vi "Argument check.vi"(8 "error in":errorcluster, 10 "Arg":string="supint->out2,12", 11 "par":string="export void vtSysPwrSupVoltSet (char vt7001CfgEntry[], float volt)") -> (0 "error out":errorcluster, 3 "Check result":string="√")   [LabVIEW 2010]
panel:
  out "Enum":T1(ring)=enum."float"
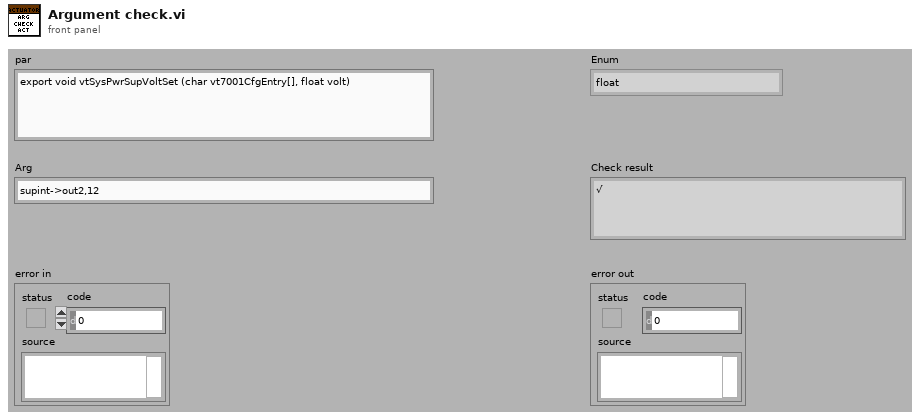
[diagram p1: front panel]
types:
  T1 = enum16{"char", "float", "double", "int", "long", "enum"}
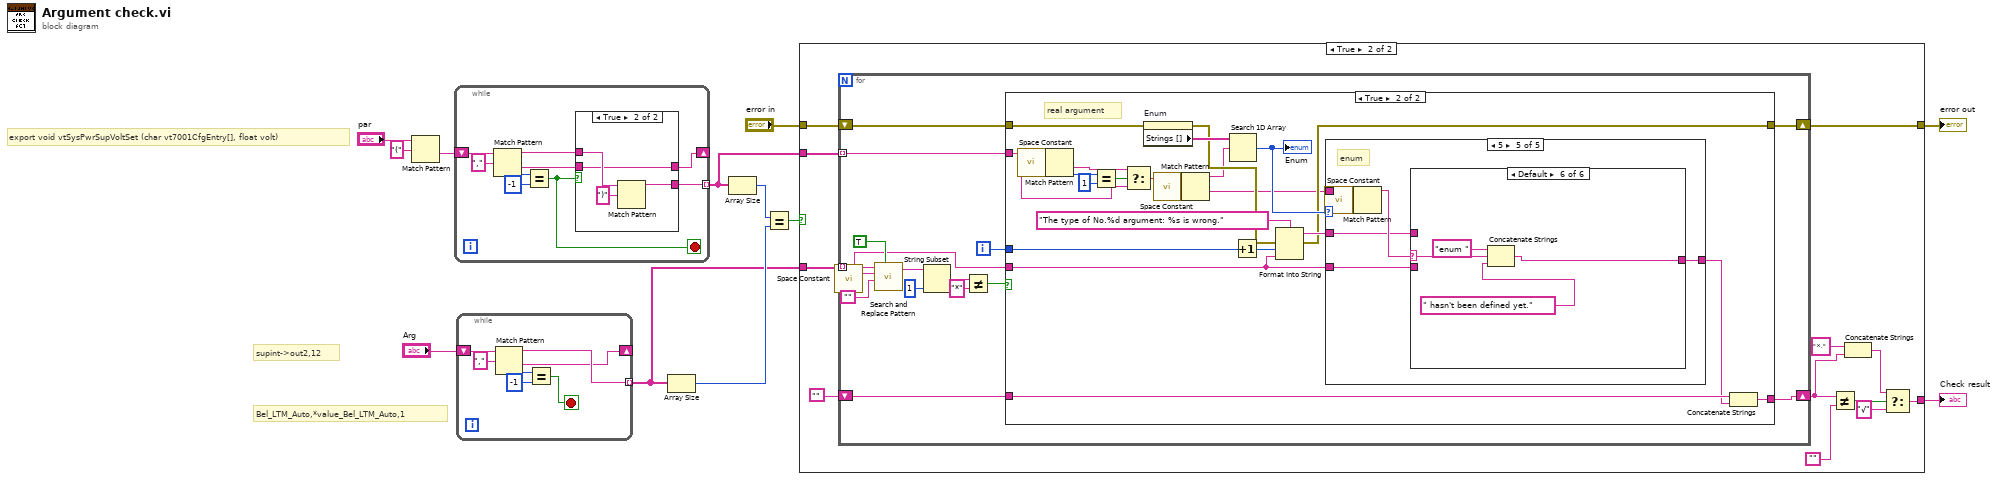
[diagram p0: block diagram]
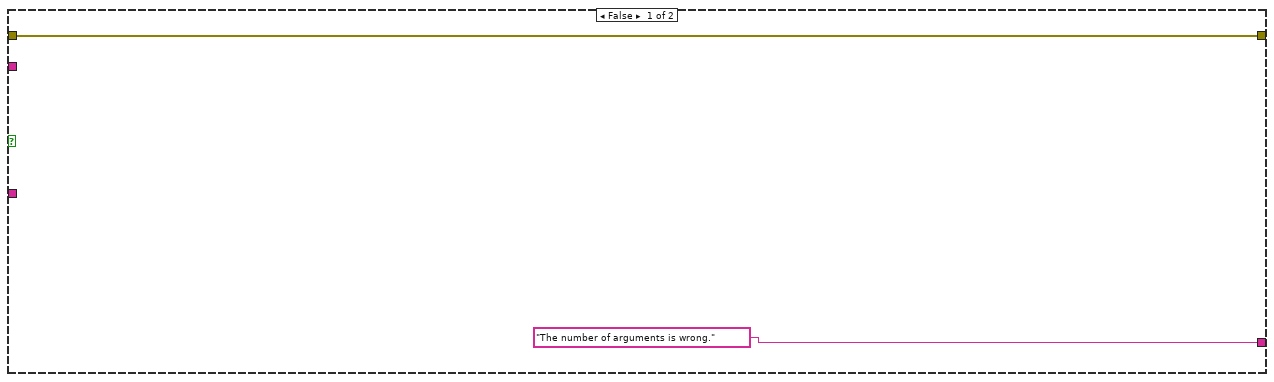
[diagram p2: hidden frame]
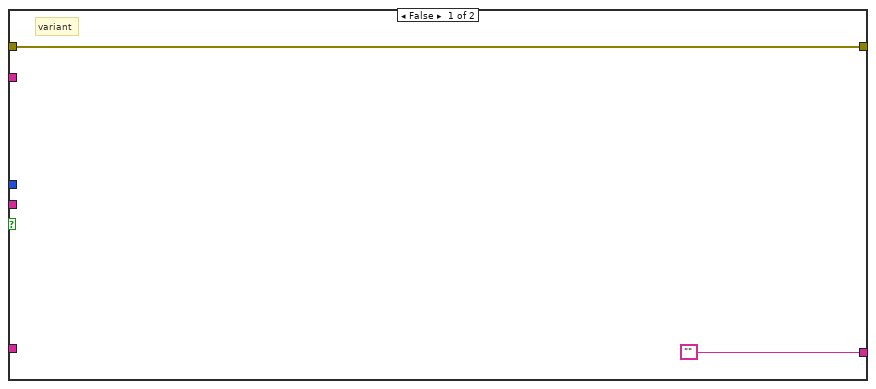
[diagram p3: hidden frame]
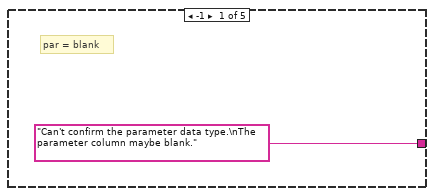
[diagram p4: hidden frame]
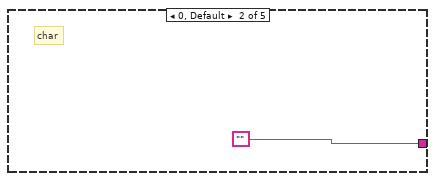
[diagram p5: hidden frame]
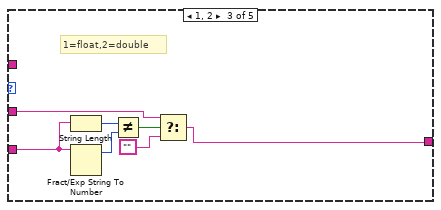
[diagram p6: hidden frame]
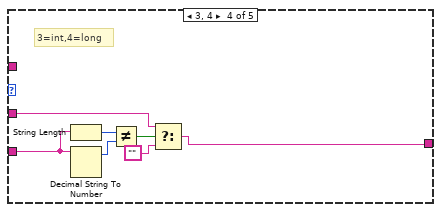
[diagram p7: hidden frame]
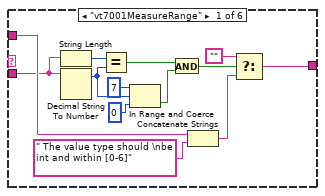
[diagram p8: hidden frame]
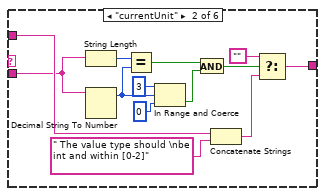
[diagram p9: hidden frame]
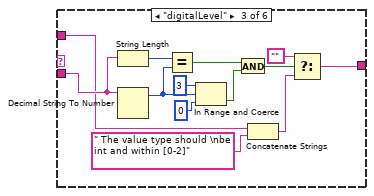
[diagram p10: hidden frame]
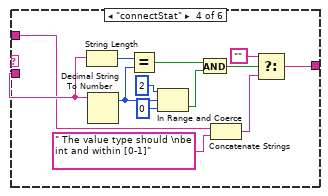
[diagram p11: hidden frame]
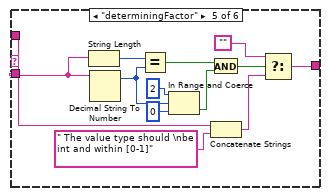
[diagram p12: hidden frame]
diagram:
  # "Bel_LTM_Auto,*value_Bel_LTM_Auto,1"
  # "supint->out2,12"
  # "export void vtSysPwrSupVoltSet (char vt7001CfgEntry[], float volt)"
  n1 = Match Pattern(string="par", regular expression="(") -> (after substring=w11:string)  [unwired: 1 in, 3 out]
  n2 = while {
    shift-right: [w14] -> _
    shift-left: w11 -> [w21]
    tunnel: [w16] -> w7 mode=indexing
    stop <- w13 stop-if-true
    n3 = Match Pattern(string=w21, regular expression=",") -> (before substring=w17:string, after substring=w15:string, offset past match=w19:i32)  [unwired: 1 in, 1 out]
    n4 = Equal?(x=w19, y=-1) -> (x = y?=w13:bool)
    n5 = case shown="True" w13 {
      tunnel: w17 -> [w23 w27]
      tunnel: [w23 w25] -> w16
      tunnel: w15 -> [w22 w24]
      tunnel: [w22 w24] -> w14
      frame False {
      }
      frame True {
        n6 = Match Pattern(string=w27, regular expression=")") -> (before substring=w25:string)  [unwired: 1 in, 3 out]
      }
    }
  }
  n7 = while {
    shift-right: [w29] -> _
    shift-left: "Arg" -> [w34]
    tunnel: [w30] -> w6 mode=indexing
    stop <- w28 stop-if-true
    n8 = Match Pattern(string=w34, regular expression=",") -> (before substring=w30:string, after substring=w29:string, offset past match=w32:i32)  [unwired: 1 in, 1 out]
    n9 = Equal?(x=w32, y=-1) -> (x = y?=w28:bool)
  }
  n10 = Array Size(array=w6) -> (size(s)=w9:i32)
  n11 = Array Size(array=w7) -> (size(s)=w10:i32)
  n12 = Equal?(x=w10, y=w9) -> (x = y?=w8:bool)
  n13 = case shown="True" w8 {
    tunnel: w7 -> [_ w48]
    tunnel: w6 -> [_ w47]
    tunnel: ["The number of arguments is wrong." w42] -> w5
    tunnel: "error in" -> [w35 w41]
    tunnel: [w35 w40] -> w2
    frame False {
    }
    frame True {
      n14 = for {
        tunnel: w48 -> [w63] mode=indexing
        tunnel: w47 -> [w49] mode=indexing
        shift-right: [w61] -> w38
        shift-left: "" -> [w62]
        shift-right: [w59] -> w40
        shift-left: w41 -> [w60]
        i -> [w50]
        n15 = call <vilib>:"Space Constant.vi"() -> ("String"=w58:string)
        n16 = call <vilib>:"Search and Replace Pattern.vi"("string"=w49, "regular expression (\"\")"=w58, "replace string (\"\")"="", "replace all? (F)"=TRUE) -> ("result string"=w55:string)  [unwired: 1 in, 1 out]
        n17 = String Subset(string=w55, length (rest)=1 ("length (rest)")) -> (substring=w53:string)  [unwired: 1 in]
        n18 = Not Equal?(x=w53, y="*") -> (x != y?=w51:bool)
        n19 = case shown="True" w51 {
          tunnel: w63 -> [_ w82]
          tunnel: w62 -> [_ w74]
          tunnel: ["" w72] -> w61
          tunnel: w60 -> [w64 w71]
          tunnel: [w64 w70] -> w59
          tunnel: w50 -> [_ w69]
          tunnel: w49 -> [_ w68]
          frame False {
            # "variant"
          }
          frame True {
            # "real argument"
            n20 = call <vilib>:"Space Constant.vi"() -> ("String"=w88:string)
            n21 = Match Pattern(string=w82, regular expression=w88) -> (after substring=w86:string, offset past match=w81:i32)  [unwired: 1 in, 2 out]
            n22 = Equal?(x=w81, y=1) -> (x = y?=w87:bool)
            n23 = Select(t=w86, s=w87, f=w82) -> (s? t:f=w83:string)
            n24 = property on="Enum" class="Enum (strict)"(error in=w71) -> (error out=w76:errorcluster, "Strings []"=w84:string[])  [unwired: 1 in, 1 out]
            n25 = call <vilib>:"Space Constant.vi"() -> ("String"=w85:string)
            n26 = Match Pattern(string=w83, regular expression=w85) -> (before substring=w67:string, after substring=w66:string)  [unwired: 1 in, 2 out]
            n27 = Search 1D Array(1D array=w84, element=w67) -> (index of element=w79:i32)  [unwired: 1 in]
            "Enum" <- w79
            n28 = Increment(x=w69) -> (x+1=w77:i32)
            n29 = Format Into String(format string="The type of No.%d argument: %s is wrong.", error in=w76, w77, w68) -> (resulting string=w75:string, error out=w70:errorcluster)  [unwired: 1 in]
            n30 = case shown="5" w79 {
              tunnel: w68 -> [_ _ w95 w104 w106]
              tunnel: w75 -> [_ _ w92 w100 w107]
              tunnel: ["Can't confirm the parameter data type.\nThe parameter column maybe blank." "" w91 w98 w105] -> w73
              tunnel: w66 -> [_ _ _ _ w110]
              frame -1 {
                # "par = blank"
              }
              frame 0, Default {
                # "char"
              }
              frame 1, 2 {
                # "1=float,2=double"
                n31 = String Length(string=w95) -> (length=w97:i32)
                n32 = Fract/Exp String To Number(string=w95) -> (offset past number=w96:i32)  [unwired: 3 in, 1 out]
                n33 = Not Equal?(x=w97, y=w96) -> (x != y?=w94:bool)
                n34 = Select(t=w92, s=w94, f="") -> (s? t:f=w91:string)
              }
              frame 3, 4 {
                # "3=int,4=long"
                n35 = String Length(string=w104) -> (length=w103:i32)
                n36 = Decimal String To Number(string=w104) -> (offset past number=w102:i32)  [unwired: 2 in, 1 out]
                n37 = Not Equal?(x=w103, y=w102) -> (x != y?=w101:bool)
                n38 = Select(t=w100, s=w101, f="") -> (s? t:f=w98:string)
              }
              frame 5 {
                # "enum"
                n39 = call <vilib>:"Space Constant.vi"() -> ("String"=w109:string)
                n40 = Match Pattern(string=w110, regular expression=w109) -> (before substring=w108:string)  [unwired: 1 in, 3 out]
                n41 = case shown="Default" w108 {
                  selector: w108 -> [_ _ _ _ _ w179]
                  tunnel: w107 -> [w113 w126 w138 w151 w164 _]
                  tunnel: w106 -> [w112 w125 w139 w152 w166 _]
                  tunnel: [w111 w124 w137 w150 w165 w177] -> w105
                  frame "vt7001MeasureRange" {
                    n42 = String Length(string=w112) -> (length=w123:i32)
                    n43 = Decimal String To Number(string=w112) -> (offset past number=w121:i32)  [unwired: 2 in, 1 out]
                    n44 = Equal?(x=w123, y=w121) -> (x = y?=w122:bool)
                    n45 = In Range and Coerce(upper limit=7, x=w121, lower limit=0) -> (In Range?=w118:bool)  [unwired: 1 out]
                    n46 = And(x=w122, y=w118) -> (x .and. y?=w117:bool)
                    n47 = Concatenate Strings(w113, " The value type should \nbe int and within [0-6]" ("string")) -> (w115:string)
                    n48 = Select(t="", s=w117, f=w115) -> (s? t:f=w111:string)
                  }
                  frame "currentUnit" {
                    n49 = String Length(string=w125) -> (length=w136:i32)
                    n50 = Decimal String To Number(string=w125) -> (offset past number=w134:i32)  [unwired: 2 in, 1 out]
                    n51 = Equal?(x=w136, y=w134) -> (x = y?=w135:bool)
                    n52 = In Range and Coerce(upper limit=3, x=w134, lower limit=0) -> (In Range?=w131:bool)  [unwired: 1 out]
                    n53 = And(x=w135, y=w131) -> (x .and. y?=w130:bool)
                    n54 = Concatenate Strings(w126, " The value type should \nbe int and within [0-2]" ("string")) -> (w128:string)
                    n55 = Select(t="", s=w130, f=w128) -> (s? t:f=w124:string)
                  }
                  frame "digitalLevel" {
                    n56 = String Length(string=w139) -> (length=w149:i32)
                    n57 = Decimal String To Number(string=w139) -> (offset past number=w147:i32)  [unwired: 2 in, 1 out]
                    n58 = Equal?(x=w149, y=w147) -> (x = y?=w148:bool)
                    n59 = In Range and Coerce(upper limit=3, x=w147, lower limit=0) -> (In Range?=w144:bool)  [unwired: 1 out]
                    n60 = And(x=w148, y=w144) -> (x .and. y?=w143:bool)
                    n61 = Concatenate Strings(w138, " The value type should \nbe int and within [0-2]" ("string")) -> (w141:string)
                    n62 = Select(t="", s=w143, f=w141) -> (s? t:f=w137:string)
                  }
                  frame "connectStat" {
                    n63 = String Length(string=w152) -> (length=w162:i32)
                    n64 = Decimal String To Number(string=w152) -> (offset past number=w160:i32)  [unwired: 2 in, 1 out]
                    n65 = Equal?(x=w162, y=w160) -> (x = y?=w161:bool)
                    n66 = In Range and Coerce(upper limit=2, x=w160, lower limit=0) -> (In Range?=w157:bool)  [unwired: 1 out]
                    n67 = And(x=w161, y=w157) -> (x .and. y?=w156:bool)
                    n68 = Concatenate Strings(w151, " The value type should \nbe int and within [0-1]" ("string")) -> (w154:string)
                    n69 = Select(t="", s=w156, f=w154) -> (s? t:f=w150:string)
                  }
                  frame "determiningFactor" {
                    n70 = String Length(string=w166) -> (length=w175:i32)
                    n71 = Decimal String To Number(string=w166) -> (offset past number=w173:i32)  [unwired: 2 in, 1 out]
                    n72 = Equal?(x=w175, y=w173) -> (x = y?=w174:bool)
                    n73 = In Range and Coerce(upper limit=2, x=w173, lower limit=0) -> (In Range?=w170:bool)  [unwired: 1 out]
                    n74 = And(x=w174, y=w170) -> (x .and. y?=w169:bool)
                    n75 = Concatenate Strings(w164, " The value type should \nbe int and within [0-1]" ("string")) -> (w163:string)
                    n76 = Select(t="", s=w169, f=w163) -> (s? t:f=w165:string)
                  }
                  frame Default {
                    n77 = Concatenate Strings("enum " ("string"), w179, " hasn't been defined yet.") -> (w177:string)
                  }
                }
              }
            }
            n78 = Concatenate Strings(w74, w73) -> (w72:string)
          }
        }
      }
      n79 = Not Equal?(x=w38, y="") -> (x != y?=w44:bool)
      n80 = Concatenate Strings("×,", w38) -> (w37:string)
      n81 = Select(t=w37, s=w44, f="√") -> (s? t:f=w42:string)
    }
  }
  "Check result" <- w5
  "error out" <- w2
